vi "Go Position.vi"(10 "Position":dbl) -> ()   [LabVIEW 2017]
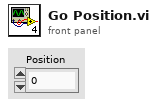
[diagram p1: front panel]
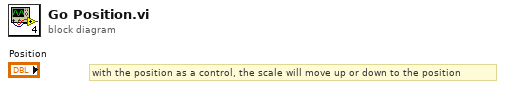
[diagram p0: block diagram]
diagram:
  # "with the position as a control, the scale will move up or down to the position"
